vi "Get_Remote_Process_List.vi"(6 "timeout (30 s)":i32=30, 8 "error in (no error)":errorcluster, 11 "IP Address or PC Name":string="CustardPie") -> (0 "error out":errorcluster, 3 "Process List (\\\\[IPAddress]\\[Process])":string[](array[string]))   [LabVIEW 2016, in "data.citadel.lvclass"]
doc: "This VI gets a list of Shared Variable Processes on a remote machine.\n\nCreated By:\nRyan Pacini\n11/31/11"
uses:
  data.citadel.lvclass
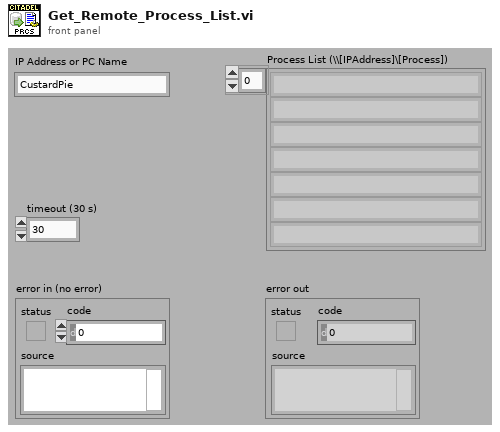
[diagram p1: front panel]
types:
  T1 = enum16{"BT_UNDEFINED", "BT_MACHINE", "BT_PROCESS", "BT_CONTROLENV", "BT_FOLDER", "BT_BLOCK", "BT_BLOCKFOLDER", "BT_ITEM", "BT_ITEMRANGE", "BT_DATABASE", "BT_OPCGROUP", "BT_LKMEMBER", "BT_MEMBER", "BT_CFGOBJECT", "BT_ALARM", "BT_MEMBERRANGE", "BT_LKMEMBERRANGE", "BT_IMPLICIT_MEMBER", "BT_FOLDER_RANGE", "BT_CFGCLASS", "BT_CFGATTR", "BT_NETHOOD", "BT_NETWORK", "BT_DOMAIN", "BT_RUN", "BT_ALARMSERVER"}
  T2 = cluster{"browseType_":enum16{"BT_UNDEFINED", "BT_MACHINE", "BT_PROCESS", "BT_CONTROLENV", "BT_FOLDER", "BT_BLOCK", "BT_BLOCKFOLDER", "BT_ITEM", "BT_ITEMRANGE", "BT_DATABASE", "BT_OPCGROUP", "BT_LKMEMBER", "BT_MEMBER", "BT_CFGOBJECT", "BT_ALARM", "BT_MEMBERRANGE", "BT_LKMEMBERRANGE", "BT_IMPLICIT_MEMBER", "BT_FOLDER_RANGE", "BT_CFGCLASS", "BT_CFGATTR", "BT_NETHOOD", "BT_NETWORK", "BT_DOMAIN", "BT_RUN", "BT_ALARMSERVER"}, "dataType_":u16, "szDelim_":string, "name_":string, "prototype_":variant, "rights_":i16, "BROWSE_FLAGS":u16}[]
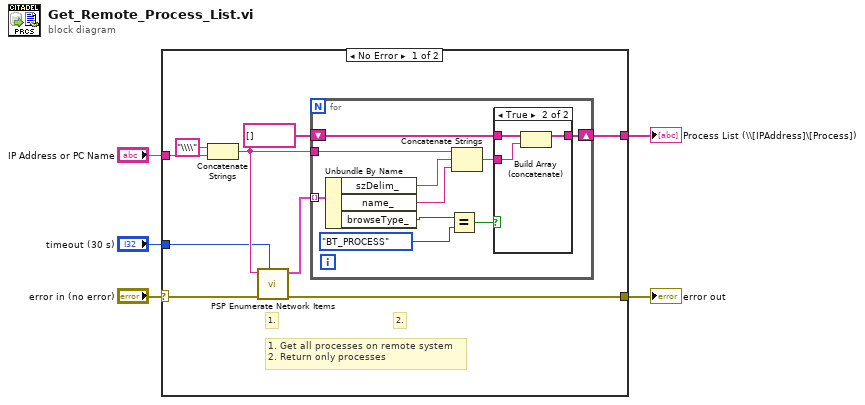
[diagram p0: block diagram]
diagram:
  n1 = case shown="No Error" "error in (no error)" {
    selector: "error in (no error)" -> [w7 w29]
    tunnel: "IP Address or PC Name" -> [w14 _]
    tunnel: [w9 _] -> w4
    tunnel: [w8 w29] -> w3
    tunnel: "timeout (30 s)" -> [w6 _]
    frame No Error {
      # "1. Get all processes on remote system\n2. Return only processes"
      # "2."
      # "1."
      n2 = Concatenate Strings("\\\\" ("string"), w14) -> (w10:string)
      n3 = call <vilib>:"PSP Enumerate Network Items.vi"("timeout (30 s)"=w6, "error in (no error)"=w7, "Browse Path"=w10) -> ("error out"=w8:errorcluster, "Items"=w12:T2)  [unwired: 7 in]
      n4 = for {
        tunnel: w12 -> [w21] mode=indexing
        shift-right: [w20] -> w9
        shift-left: string[] [] -> [w19]
        tunnel: w10 -> [w18]
        n5 = Unbundle By Name(w21) -> ("szDelim_"=w17:string, "name_"=w16:string, "browseType_"=w24:T1)
        n6 = Equal?(x=w24, y=T1."BT_PROCESS" ("browseType_")) -> (x = y?=w22:bool)
        n7 = Concatenate Strings(w18, w17, w16) -> (w15:string)
        n8 = case shown="True" w22 {
          tunnel: [w25 w28] -> w20
          tunnel: w19 -> [w25 w27]
          tunnel: w15 -> [_ w26]
          frame False {
          }
          frame True {
            n9 = Build Array (concatenate)(w27, w26) -> (w28:string[])
          }
        }
      }
    }
    frame Error {
    }
  }
  "Process List (\\\\[IPAddress]\\[Process])" <- w4
  "error out" <- w3
